vi "AudioAnalysis.vi"() -> ()   [LabVIEW 2014]
uses:
  <vilib>/express/express analysis/Spectral/Block/exnSpectralBlock spectral measurements RMS poly.vi
  <vilib>/express/express analysis/Spectral/Block/exnSpectralBlock spectral measurements RMS DDT.vi
  <vilib>/express/express analysis/Spectral/XNode/ExpressSpectralMeasurementsBlockNode.xnode
panel:
  in  "Frequency":dbl=10.0
  out "Array":dbl[](array[numeric])
  in  "stop":bool
  out "Waveform Graph 3":dynamicdata(graph)
  out "Waveform Graph":dynamicdata(graph)
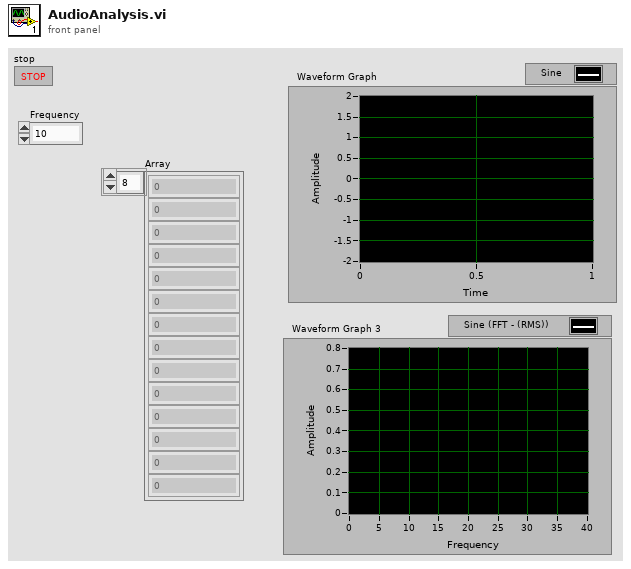
[diagram p1: front panel]
types:
  T1 = cluster{"averaging mode":u16, "weighting mode":u16, "number of averages":u32}
  T2 = cluster{"dB On (F)":bool, "unwrap phase (F)":bool, "convert to degree (F)":bool}
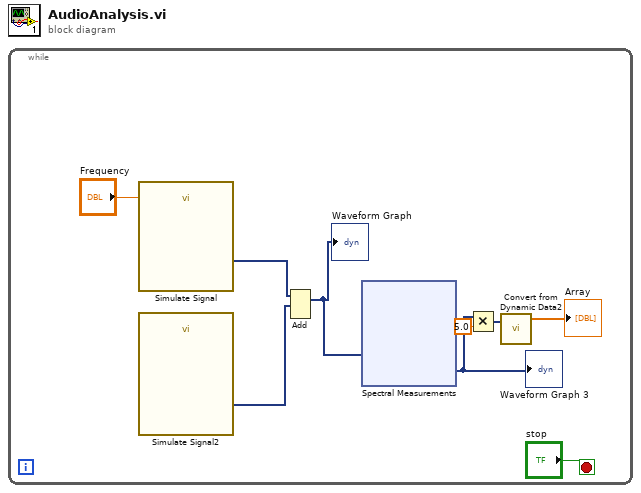
[diagram p0: block diagram]
diagram:
  n1 = while {
    stop <- "stop" stop-if-true
    n2 = call "Simulate Signal"("Frequency"="Frequency") -> ("Sine"=w7:dynamicdata)  [unwired: 13 in, 1 out]
    n3 = call "Simulate Signal2"() -> ("Sine"=w9:dynamicdata)  [unwired: 14 in, 1 out]
    n4 = Add(1:w9, 2:w7) -> (0:w8:dynamicdata)  [unwired: 1 in, 1 out]
    "Waveform Graph" <- w8
    n5 = xnode "Spectral Measurements"("Signals"=w8) -> ("FFT - (RMS)"=w5:dynamicdata)  [unwired: 1 in, 2 out]
    "Waveform Graph 3" <- w5
    n6 = Multiply(x=w5, y=5.0) -> (x*y=w2:dynamicdata)
    n7 = call "Convert from Dynamic Data2"("Dynamic Data Type"=w2) -> ("Array"=→"Array":dbl[])  [unwired: 3 in]
  }
